vi "Reserve (N Sessions).vi"(6 "timeout in milliseconds":i32, 8 "error in":errorcluster, 9 "instrument type ID":string, 10 "pin or relay names":string[](array[string]), 11 "Measurement Context In":refnum<class "Measure Call Context.lvclass">) -> (0 "error out":errorcluster, 1 "gRPC clients out":T1, 2 "session information":T3[](array[typedef]), 3 "Measurement Context out":refnum<class "Measure Call Context.lvclass">)   [LabVIEW 2020, in "Measurement Service Helpers.lvlib"]
doc: "Reserves sessions based on the provided pin information."
uses:
  Measurement Service Helpers.lvlib
  <vilib>/MeasurementLink/MeasurementLink Discovery Client/MeasurementLink Discovery Client.lvlib
  <vilib>/MeasurementLink/MeasurementLink Session Management Client/MeasurementLink Session Management Client.lvlib
  <vilib>/MeasurementLink/MeasurementLink Discovery Client/RPC Messages/ni_measurementlink_discovery_v1_ResolveServiceRequest.ctl
  <vilib>/MeasurementLink/MeasurementLink Session Management Client/RPC Messages/ni_measurementlink_PinMapContext.ctl
  <vilib>/MeasurementLink/MeasurementLink Session Management Client/RPC Messages/ni_measurementlink_sessionmanagement_v1_ReserveSessionsRequest.ctl
  <vilib>/gRPC/LabVIEW gRPC Library/Shared/grpcId.ctl
  <vilib>/gRPC/LabVIEW gRPC Library/grpc-lvsupport-release.lvlib
  GRPC Clients.ctl
  <vilib>/MeasurementLink/MeasurementLink Measurement Server/Measure Call Context/Measure Call Context.lvclass
  <vilib>/MeasurementLink/MeasurementLink Session Management Client/RPC Messages/ni_measurementlink_sessionmanagement_v1_ChannelMapping.ctl
  <vilib>/MeasurementLink/MeasurementLink Session Management Client/RPC Messages/nidevice_grpc_Session.ctl
  <vilib>/MeasurementLink/MeasurementLink Session Management Client/RPC Messages/ni_measurementlink_sessionmanagement_v1_SessionInformation.ctl
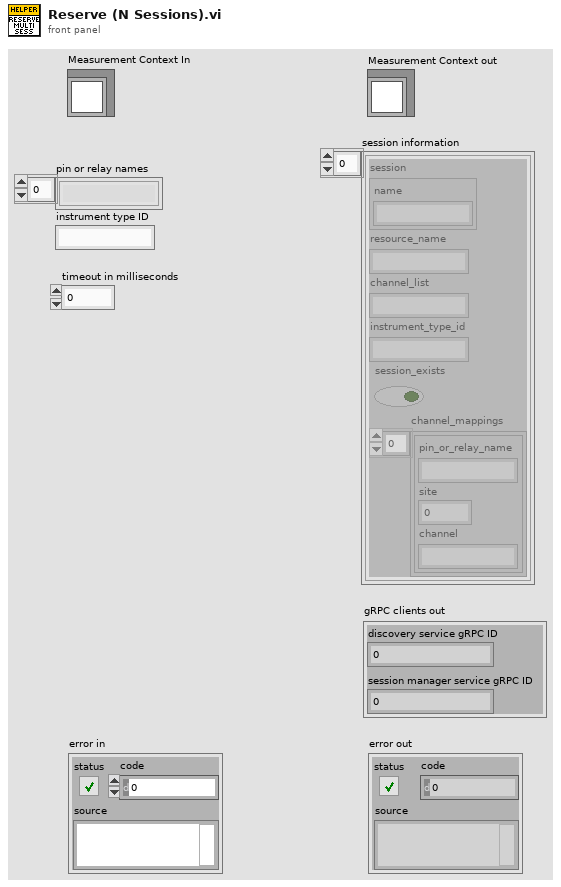
[diagram p1: front panel]
types:
  T1 = typedef "Measurement Service Helpers.lvlib/GRPC Clients.ctl" = cluster{"discovery service gRPC ID":T2, "session manager service gRPC ID":T2}
  T2 = typedef "grpc-lvsupport-release.lvlib/grpcId.ctl" = u64
  T3 = typedef "MeasurementLink Session Management Client.lvlib/ni_measurementlink_sessionmanagement_v1_SessionInformation.ctl" = cluster{"session":T4, "resource_name":string, "channel_list":string, "instrument_type_id":string, "session_exists":bool, "channel_mappings":T5[]}
  T4 = typedef "MeasurementLink Session Management Client.lvlib/nidevice_grpc_Session.ctl" = cluster{"name":string}
  T5 = typedef "MeasurementLink Session Management Client.lvlib/ni_measurementlink_sessionmanagement_v1_ChannelMapping.ctl" = cluster{"pin_or_relay_name":string, "site":i32, "channel":string}
  T6 = typedef "MeasurementLink Session Management Client.lvlib/ni_measurementlink_sessionmanagement_v1_ReserveSessionsRequest.ctl" = cluster{"pin_map_context":T7, "pin_or_relay_names":string[], "instrument_type_id":string, "timeout_in_milliseconds":i32}
  T7 = typedef "MeasurementLink Session Management Client.lvlib/ni_measurementlink_PinMapContext.ctl" = cluster{"pin_map_id":string, "sites":i32[]}
  T8 = typedef "MeasurementLink Discovery Client.lvlib/ni_measurementlink_discovery_v1_ResolveServiceRequest.ctl" = cluster{"provided_interface":string, "service_class":string}
  T9 = typedef "MeasurementLink Measurement Server.lvlib/PinMapContext.ctl" = cluster{"pin_map_id":string, "sites":i32[]}
  T10 = typedef "MeasurementLink Discovery Client.lvlib/ni_measurementlink_discovery_v1_ServiceLocation.ctl" = cluster{"location":string, "insecure_port":string, "ssl_authenticated_port":string}
  T11 = typedef "MeasurementLink Session Management Client.lvlib/ni_measurementlink_sessionmanagement_v1_ReserveSessionsResponse.ctl" = cluster{"sessions":T3[]}
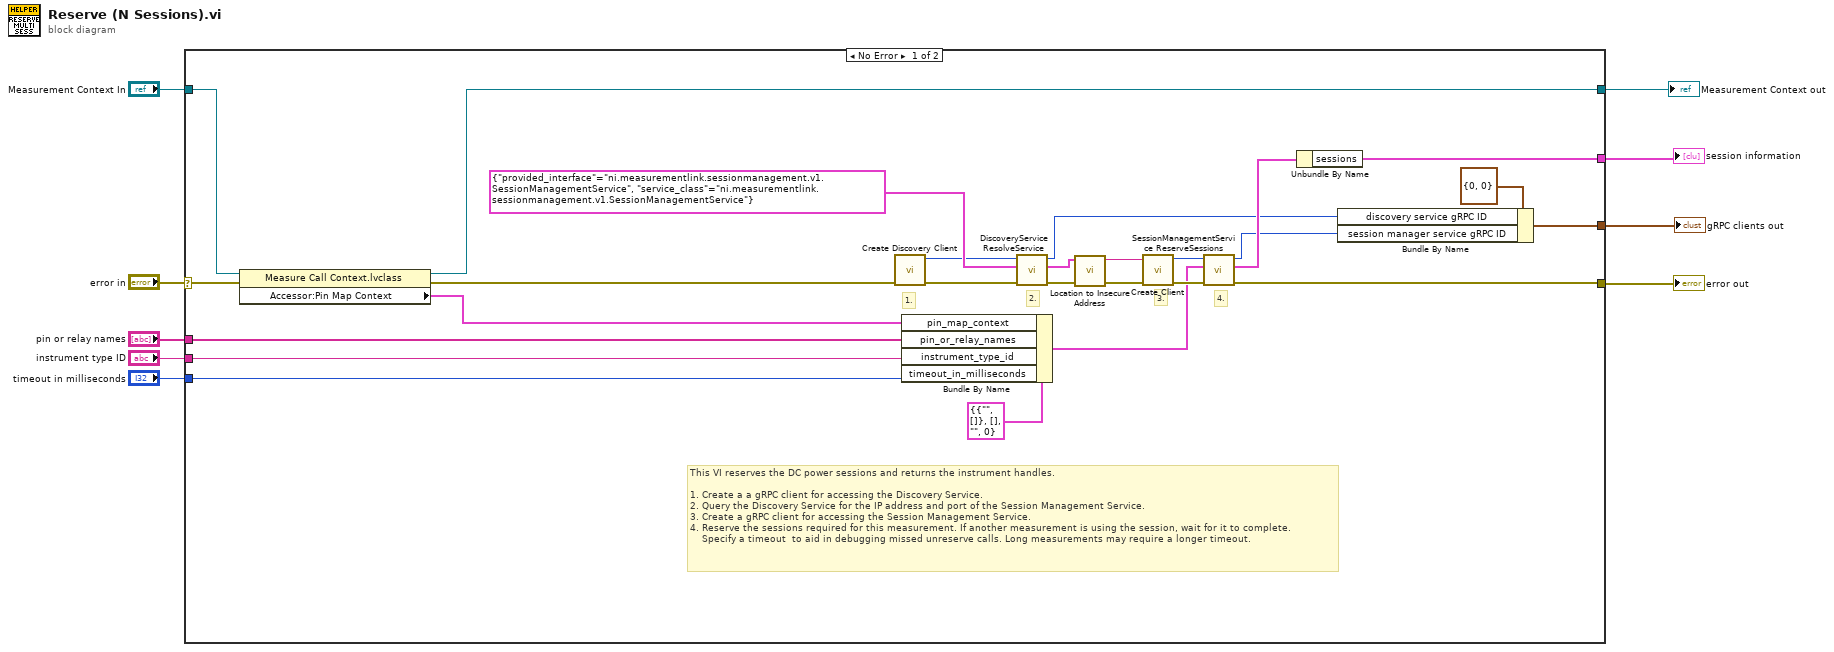
[diagram p0: block diagram]
diagram:
  n1 = case shown="No Error" "error in" {
    selector: "error in" -> [w13 w36]
    tunnel: [w31 w36] -> w9
    tunnel: "instrument type ID" -> [w27 _]
    tunnel: "timeout in milliseconds" -> [w26 _]
    tunnel: "pin or relay names" -> [w24 _]
    tunnel: [w23 _] -> w5
    tunnel: [w18 _] -> w4
    tunnel: "Measurement Context In" -> [w16 w35]
    tunnel: [w14 w35] -> w2
    frame No Error {
      # "4."
      # "3."
      # "2."
      # "1."
      # "This VI reserves the DC power sessions and returns the instrument handles.\n\n1. Create a a gRPC client for accessing the Discovery Service.\n2. Query the Discovery Service for the IP address and port of the Session Management Service.\n3. Create a gRPC client for accessing the Session Management Service.\n4. Reserve the sessions required for this measurement. If another measurement is using the session, wait for it to complete. \n    Specify a timeout  to aid in debugging missed unreserve calls. Long measurements may require a longer timeout."
      n2 = property class="Measure Call Context.lvclass"(reference=w16, error in=w13) -> (reference out=w14:refnum<class "Measure Call Context.lvclass">, error out=w17:errorcluster, "Accessor:Pin Map Context"=w15:T9)
      n3 = call "Create Discovery Client.vi"("error in"=w17) -> ("error out"=w12:errorcluster, "discovery service gRPC ID Out"=w11:T2)  [unwired: 9 in]
      n4 = Bundle By Name(cluster=T6 {"pin_map_context"={"pin_map_id"="", "sites"=[]}, "pin_or_relay_names"=[], "instrument_type_id"="", "timeout_in_milliseconds"=0} ("Request Data"), "pin_map_context"=w15, "pin_or_relay_names"=w24, "instrument_type_id"=w27, "timeout_in_milliseconds"=w26) -> (w25:T6)
      n5 = call <vilib>:"DiscoveryService ResolveService.vi"("error in"=w12, "Request Data"=T8 {"provided_interface"="ni.measurementlink.sessionmanagement.v1.SessionManagementService", "service_class"="ni.measurementlink.sessionmanagement.v1.SessionManagementService"}, "gRPC ID"=w11) -> ("error out"=w32:errorcluster, "Response Data"=w22:T10, "gRPC ID out"=w10:T2)  [unwired: 6 in]
      n6 = call "Location to Insecure Address.vi"("Location"=w22) -> ("String"=w21:string)  [unwired: 10 in]
      n7 = call <vilib>:"Create Client.vi"("error in"=w32, "address"=w21) -> ("error out"=w33:errorcluster, "gRPC ID Out"=w34:T2)  [unwired: 8 in]
      n8 = call <vilib>:"SessionManagementService ReserveSessions.vi"("error in"=w33, "Request Data"=w25, "gRPC ID"=w34) -> ("error out"=w31:errorcluster, "Response Data"=w29:T11, "gRPC ID out"=w20:T2)  [unwired: 6 in]
      n9 = Unbundle By Name(w29) -> ("sessions"=w23:T3[])
      n10 = Bundle By Name(cluster=T1 {"discovery service gRPC ID"=0, "session manager service gRPC ID"=0} ("gRPC channel pool out"), "discovery service gRPC ID"=w10, "session manager service gRPC ID"=w20) -> (w18:T1)
    }
    frame Error {
    }
  }
  "error out" <- w9
  "session information" <- w5
  "gRPC clients out" <- w4
  "Measurement Context out" <- w2
